vi "Connect.vi"(8 "error in (no error)":errorcluster, 10 "Connection list in":string, 11 "Consumer in":refnum<class "Consumer.lvclass">) -> (0 "error out":errorcluster, 3 "Consumer out":refnum<class "Consumer.lvclass">)   [LabVIEW 2017, in "%DEVICE% Messaging.lvlib" / "Consumer.lvclass"]
uses:
  Consumer.lvclass
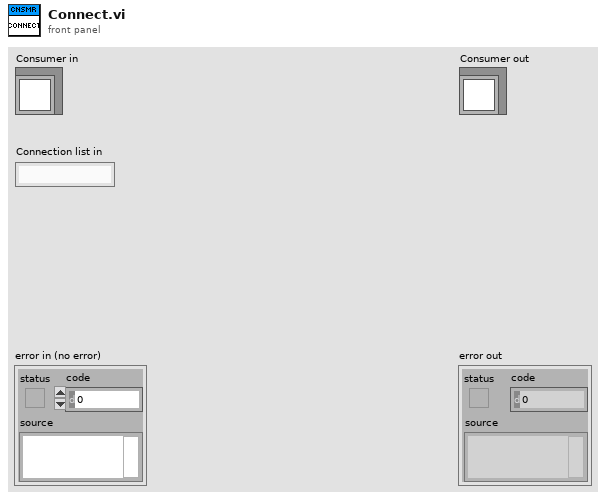
[diagram p1: front panel]
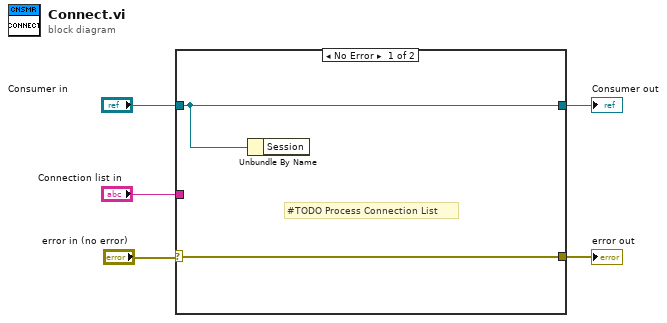
[diagram p0: block diagram]
diagram:
  n1 = case shown="No Error" "error in (no error)" {
    selector: "error in (no error)" -> [w6 w9]
    tunnel: [w6 w9] -> w4
    tunnel: [w7 w8] -> w1
    tunnel: "Consumer in" -> [w7 w8]
    tunnel: "Connection list in" -> [_ _]
    frame No Error {
      # "#TODO Process Connection List"
      n2 = Unbundle By Name(w7) -> ()  [unwired: 1 out]
    }
    frame Error {
    }
  }
  "error out" <- w4
  "Consumer out" <- w1
